vi "create solid ref image.vi"(9 "Pixel Value (default 255)":sgl=255.0, 10 "Y resolution":i32, 11 "X resolution":i32 min=0) -> (0 "error out":errorcluster, 3 "solid image":T1)   [LabVIEW 2025]
uses:
  <vilib>/vision/Image Controls.llb/IMAQ Image.ctl
  <vilib>/vision/NI_Vision_Development_Module.lvlib
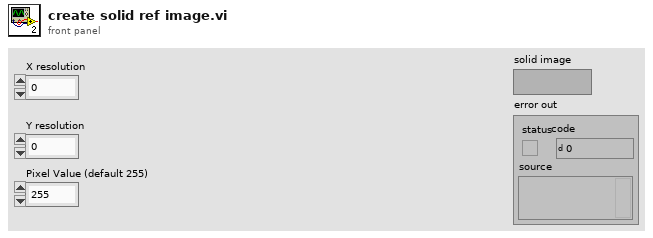
[diagram p1: front panel]
types:
  T1 = typedef "IMAQ Image.ctl" = refnum<image>
  T2 = typedef "Image Type" = u32
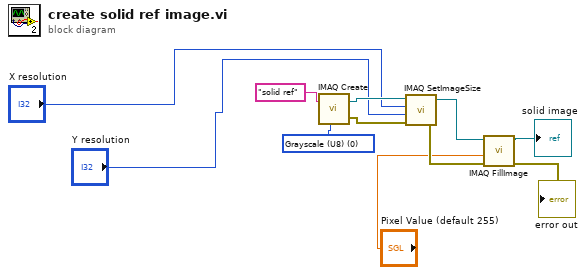
[diagram p0: block diagram]
diagram:
  w10 = T2 0 items=["Grayscale (U8)", "Grayscale (I16)", "Grayscale (SGL)", "Complex (CSG)", "RGB (U32)", "HSL (U32)", "RGB (U64)", "Grayscale (U16)"] ("Image Type")
  n1 = call "IMAQ Create"("Image Name"="solid ref", "Image Type"=w10) -> ("New Image"=w5:T1, "error out"=w9:errorcluster)  [unwired: 3 in]
  n2 = call "IMAQ SetImageSize"("error in (no error)"=w9, "Y Resolution"="Y resolution", "X Resolution"="X resolution", "Image"=w5) -> ("error out"=w8:errorcluster, "Image Out"=w2:T1)  [unwired: 1 in]
  n3 = call "IMAQ FillImage"("error in (no error)"=w8, "Pixel Value (U8, U16, I16, Float)"="Pixel Value (default 255)", "Image"=w2) -> ("error out"=→"error out":errorcluster, "Image Out"=→"solid image":T1)  [unwired: 7 in]
